vi "Login Validation (SubVI).vi"(11 "String":string) -> ()   [LabVIEW 2023]
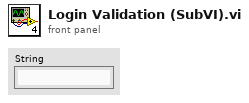
[diagram p1: front panel]
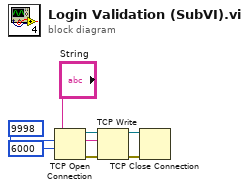
[diagram p0: block diagram]
diagram:
  n1 = TCP Open Connection(remote port or service name=u16 9998, timeout ms (60000)=6000) -> (connection ID=w1:refnum<k5>, error out=w3:errorcluster)  [unwired: 3 in]
  n2 = TCP Write(connection ID=w1, data in="String", error in (no error)=w3) -> (connection ID out=w2:refnum<k5>, error out=w4:errorcluster)  [unwired: 1 in, 1 out]
  n3 = TCP Close Connection(connection ID=w2, error in (no error)=w4) -> ()  [unwired: 1 in, 2 out]
